vi "KMultilevel Ring Test.vi"() -> ()   [LabVIEW 2015]
uses:
  KMultilevel Ring/KMultilevel Ring.xctl
panel:
  in  "stop":bool
  in  "KMultilevel Ring":string(xcontrol)
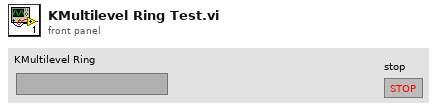
[diagram p1: front panel]
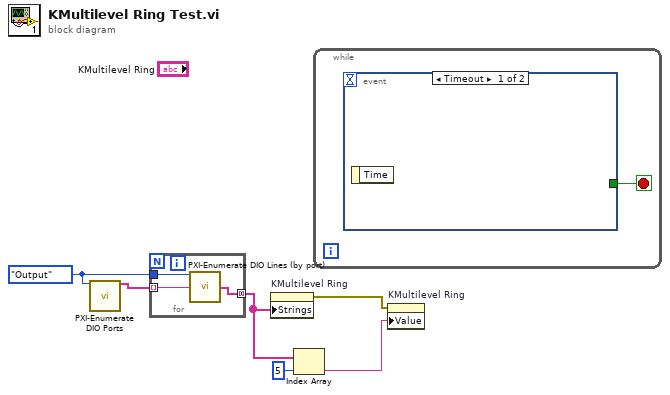
[diagram p0: block diagram]
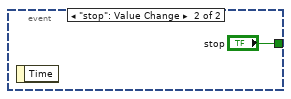
[diagram p2: hidden frame]
diagram:
  w6 = enum16{"Input", "Output"}."Output" ("Direction")
  n1 = call "PXI-Enumerate DIO Ports.vi"("Direction"=w6) -> ("Ports"=w4:tag[])  [unwired: 13 in, 1 out]
  n2 = for {
    tunnel: w4 -> [w8] mode=indexing
    tunnel: w6 -> [w9]
    tunnel: [w7] -> w2 mode=concatenating
    n3 = call "PXI-Enumerate DIO Lines (by port).vi"("Direction"=w9, "Port"=w8) -> ("Dev/Port/Lines"=w7:tag[])  [unwired: 11 in, 2 out]
  }
  n4 = property on="KMultilevel Ring" class="KMultilevel Ring (strict)"("Strings"=w2) -> (error out=w5:errorcluster)  [unwired: 2 in, 1 out]
  n5 = Index Array(array=w2, index=5) -> (element=w1:tag)
  n6 = while {
    stop <- w10 stop-if-true
    n7 = event shown="[0] Timeout" {
      selector: _ -> [_ _]
      dyn-events: _ -> [_ _]
      timeout: _ -> [_ _]
      tunnel: [_ "stop"] -> w10
      event Timeout {
        n8 = event-data() -> ()  [unwired: 1 in, 1 out]
      }
      event "stop": Value Change {
        n9 = event-data() -> ()  [unwired: 1 in, 1 out]
      }
    }
  }
  n10 = property on="KMultilevel Ring" class="KMultilevel Ring (strict)"(error in=w5, "Value"=w1) -> ()  [unwired: 1 in, 2 out]
